vi "RMX410x Configuration.vi"() -> ()   [LabVIEW 2019]
uses:
  <vilib>/addons/VeriStand Custom Device Scripting APIs/Instrument Addon/Libraries Directory/Protocols.lvlibp/RS-xxx/RS-xxx Settings.ctl
  <vilib>/addons/VeriStand Custom Device Scripting APIs/Instrument Addon/API/TypeDefs/Message Settings.ctl
  <vilib>/addons/VeriStand Custom Device Scripting APIs/Instrument Addon/API/TypeDefs/Protection Types.ctl
  <vilib>/NI VeriStand/Custom Device API/Custom Device Item Ref.ctl
  <vilib>/addons/VeriStand Custom Device Scripting APIs/Instrument Addon/API/TypeDefs/Single Channel Enumerated List Settings.ctl
  <vilib>/addons/VeriStand Custom Device Scripting APIs/Instrument Addon/API/TypeDefs/Single Channel Format Settings.ctl
  <vilib>/addons/VeriStand Custom Device Scripting APIs/Instrument Addon/API/TypeDefs/Command Settings.ctl
  <vilib>/addons/VeriStand Custom Device Scripting APIs/Instrument Addon/API/TypeDefs/Padding.ctl
  <vilib>/addons/VeriStand Custom Device Scripting APIs/Instrument Addon/API/TypeDefs/ByteCount Response Settings.ctl
  <vilib>/addons/VeriStand Custom Device Scripting APIs/Instrument Addon/API/TypeDefs/Linked Channel.ctl
  <vilib>/addons/VeriStand Custom Device Scripting APIs/Instrument Addon/API/Messages/Create Message - Periodic & Trigger.vi
  <vilib>/addons/VeriStand Custom Device Scripting APIs/Instrument Addon/API/Messages/Configure Response - Byte Count.vi
  <vilib>/addons/VeriStand Custom Device Scripting APIs/Instrument Addon/API/Messages/Create Message - Value Change & Trigger.vi
  <vilib>/addons/VeriStand Custom Device Scripting APIs/Instrument Addon/API/Channels/Create MetaData Channel - Single Channel - Format.vi
  <vilib>/addons/VeriStand Custom Device Scripting APIs/Instrument Addon/API/Channels/Create MetaData Channel - Single Channel - Enumerated List.vi
  <vilib>/addons/VeriStand Custom Device Scripting APIs/Instrument Addon/API/Channels/Create Data Channel - Single Channel - Enumerated List.vi
  <vilib>/addons/VeriStand Custom Device Scripting APIs/Instrument Addon/API/Custom Device/RS-xxx Factory.vi
  <vilib>/addons/VeriStand Custom Device Scripting APIs/Instrument Addon/API/Channels/Create Data Channel - Single Channel - Format.vi
  <vilib>/addons/VeriStand Custom Device Scripting APIs/Instrument Addon/API/Instrument Addon Scripting API.lvlib
  <vilib>/addons/VeriStand Custom Device Scripting APIs/Instrument Addon/Libraries Directory/Protocols.lvlibp/RS-xxx/RS-xxx.lvclass
  <vilib>/NI VeriStand/Custom Device API/Custom Device API.lvlib
panel:
  in  "Output System Definition File":path=path "System Definition Files/RMX410x Scripted.nivssdf"
  in  "Input System Definition File":path=path "System Definition Files/Base.nivssdf"
  # "Overview: Creates an Instrument Addon Custom Device and adds the messages and channels used to operate the NI RMX410x Rackmount Programmable DC Power Supply.\n\nThe VI executes the following steps:\n1. Creates a new Instrument Addon in the target system definition file with an RS-xxx protocol type.\n2. Creates Configuration, Control, and Feedback groups.\n3. Configures messages with created MetaData and Data Channels.\n4. Configures the messages for controlling and getting feedback from the RMX410x device.\n5. Configures the channels that control the output state and voltage levels.\n\nInstructions:\n1. Browse to the system definition file to be used as input.\n2. Browse to a path to save the system definition file as output. This may be the same as the input file.\n3. Run the VI and verify its results. \n\nFor more information on the RMX410x, refer to the RMX410x User manual:\nhttps://www.ni.com/pdf/manuals/377396c.pdf)"
  # "System Definition Files"
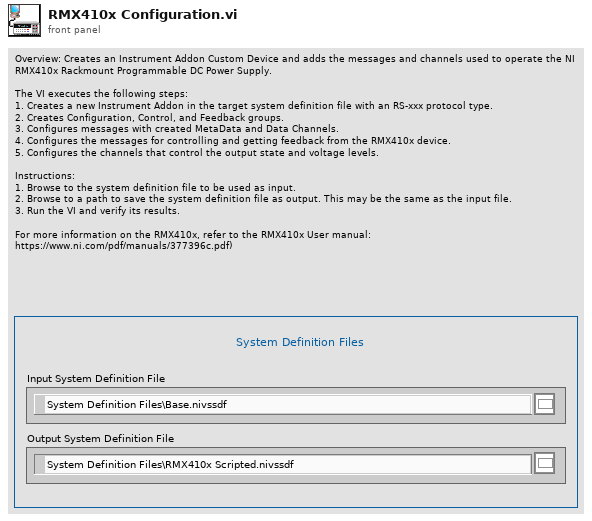
[diagram p1: front panel]
types:
  T1 = typedef "Instrument Addon Scripting API.lvlib/Linked Channel.ctl" = cluster{"Variable Name":string, "Channel Refnum":T2}
  T2 = typedef "Custom Device API.lvlib/Custom Device Item Ref.ctl" = u64
  T3 = typedef "Instrument Addon Scripting API.lvlib/ByteCount Response Settings.ctl" = cluster{"Response Format":string, "Linked Channels":T1[], "Byte Count":i32, "Use Byte Count channel":bool, "Channel Refnum":T2}
  T4 = typedef "Instrument Addon Scripting API.lvlib/Single Channel Format Settings.ctl" = cluster{"Format String":string, "Default Value":dbl, "Units":string}
  T5 = typedef "Instrument Addon Scripting API.lvlib/Single Channel Enumerated List Settings.ctl" = cluster{"Enumerated List":string[], "Default Value":dbl, "Units":string}
  T6 = cluster{"Variable Name":string, "Channel Ref in":T2}
  T7 = typedef "Instrument Addon Scripting API.lvlib/Command Settings.ctl" = cluster{"Command Format":string, "Linked Channels":cluster{"Variable Name":string, "Channel Ref in":T2}[], "Use Padding?":bool, "Padding":T8}
  T8 = typedef "Instrument Addon Scripting API.lvlib/Padding.ctl" = cluster{"Pad Value":u8, "Length":u32}
  T9 = typedef "Instrument Addon Scripting API.lvlib/Protection Types.ctl" = enum16{"None", "CRC-32", "Checksum U16", "Checksum U32", "Checksum U8"}
  T10 = typedef "Instrument Addon Scripting API.lvlib/Message Settings.ctl" = cluster{"Protection":T9, "Enable Periodic Default":bool, "Trigger Channel refnum":u64}
  T11 = enum16{"NUL", "SOH", "STX", "ETX", "EOT", "ENQ", "ACK", "BEL", "BS", "HT", "LF", "VT", "FF", "CR", "SO", "SI", "DLE", "DC1", "DC2", "DC3", "DC4", "NAK", "SYN", "ETB", "CAN", "EM", "SUB", "ESC", "FS", "GS", "RS", "US", "SP", "!", "\"", "#", "$", "%", "&", "'", "(", ")", "*", "+", ",", "- (-)", ".", "/", "0", "1", "2", "3", "4", "5", "6", "7", "8", "9", ":", ";", "<", "=", ">", "?", "@", "A", "B", "C", "D", "E", "F", "G", "H", "I", "J", "K", "L", "M", "N", "O", "P", "Q", "R", "S", "T", "U", "V", "W", "X", "Y", "Z", "[", "\\", "]", "^", "_", "`", "a", "b", "c", "d", "e", "f", "g", "h", "i", "j", "k", "l", "m", "n", "o", "p", "q", "r", "s", "t", "u", "v", "w", "x", "y", "z", "{", "|", "}", "~"}
  T12 = typedef "Protocols.lvlibp/RS-xxx.lvclass/RS-xxx Settings.ctl" = cluster{"Port":string, "Baud Rate":u32, "Data Bits":u16, "Parity":enum16{"None", "Odd", "Even", "Mark", "Space"}, "Stop Bits":u16, "Flow Control":u16, "XON":enum16{"NUL", "SOH", "STX", "ETX", "EOT", "ENQ", "ACK", "BEL", "BS", "HT", "LF", "VT", "FF", "CR", "SO", "SI", "DLE", "DC1", "DC2", "DC3", "DC4", "NAK", "SYN", "ETB", "CAN", "EM", "SUB", "ESC", "FS", "GS", "RS", "US", "SP", "!", "\"", "#", "$", "%", "&", "'", "(", ")", "*", "+", ",", "- (-)", ".", "/", "0", "1", "2", "3", "4", "5", "6", "7", "8", "9", ":", ";", "<", "=", ">", "?", "@", "A", "B", "C", "D", "E", "F", "G", "H", "I", "J", "K", "L", "M", "N", "O", "P", "Q", "R", "S", "T", "U", "V", "W", "X", "Y", "Z", "[", "\\", "]", "^", "_", "`", "a", "b", "c", "d", "e", "f", "g", "h", "i", "j", "k", "l", "m", "n", "o", "p", "q", "r", "s", "t", "u", "v", "w", "x", "y", "z", "{", "|", "}", "~"}, "XOFF":enum16{"NUL", "SOH", "STX", "ETX", "EOT", "ENQ", "ACK", "BEL", "BS", "HT", "LF", "VT", "FF", "CR", "SO", "SI", "DLE", "DC1", "DC2", "DC3", "DC4", "NAK", "SYN", "ETB", "CAN", "EM", "SUB", "ESC", "FS", "GS", "RS", "US", "SP", "!", "\"", "#", "$", "%", "&", "'", "(", ")", "*", "+", ",", "- (-)", ".", "/", "0", "1", "2", "3", "4", "5", "6", "7", "8", "9", ":", ";", "<", "=", ">", "?", "@", "A", "B", "C", "D", "E", "F", "G", "H", "I", "J", "K", "L", "M", "N", "O", "P", "Q", "R", "S", "T", "U", "V", "W", "X", "Y", "Z", "[", "\\", "]", "^", "_", "`", "a", "b", "c", "d", "e", "f", "g", "h", "i", "j", "k", "l", "m", "n", "o", "p", "q", "r", "s", "t", "u", "v", "w", "x", "y", "z", "{", "|", "}", "~"}, "End Read on Termination Character":bool, "End Write on Termination Character":bool, "Termination Character":u8}
  T13 = cluster{"Variable Name":string, "Channel Ref in":T2}[]
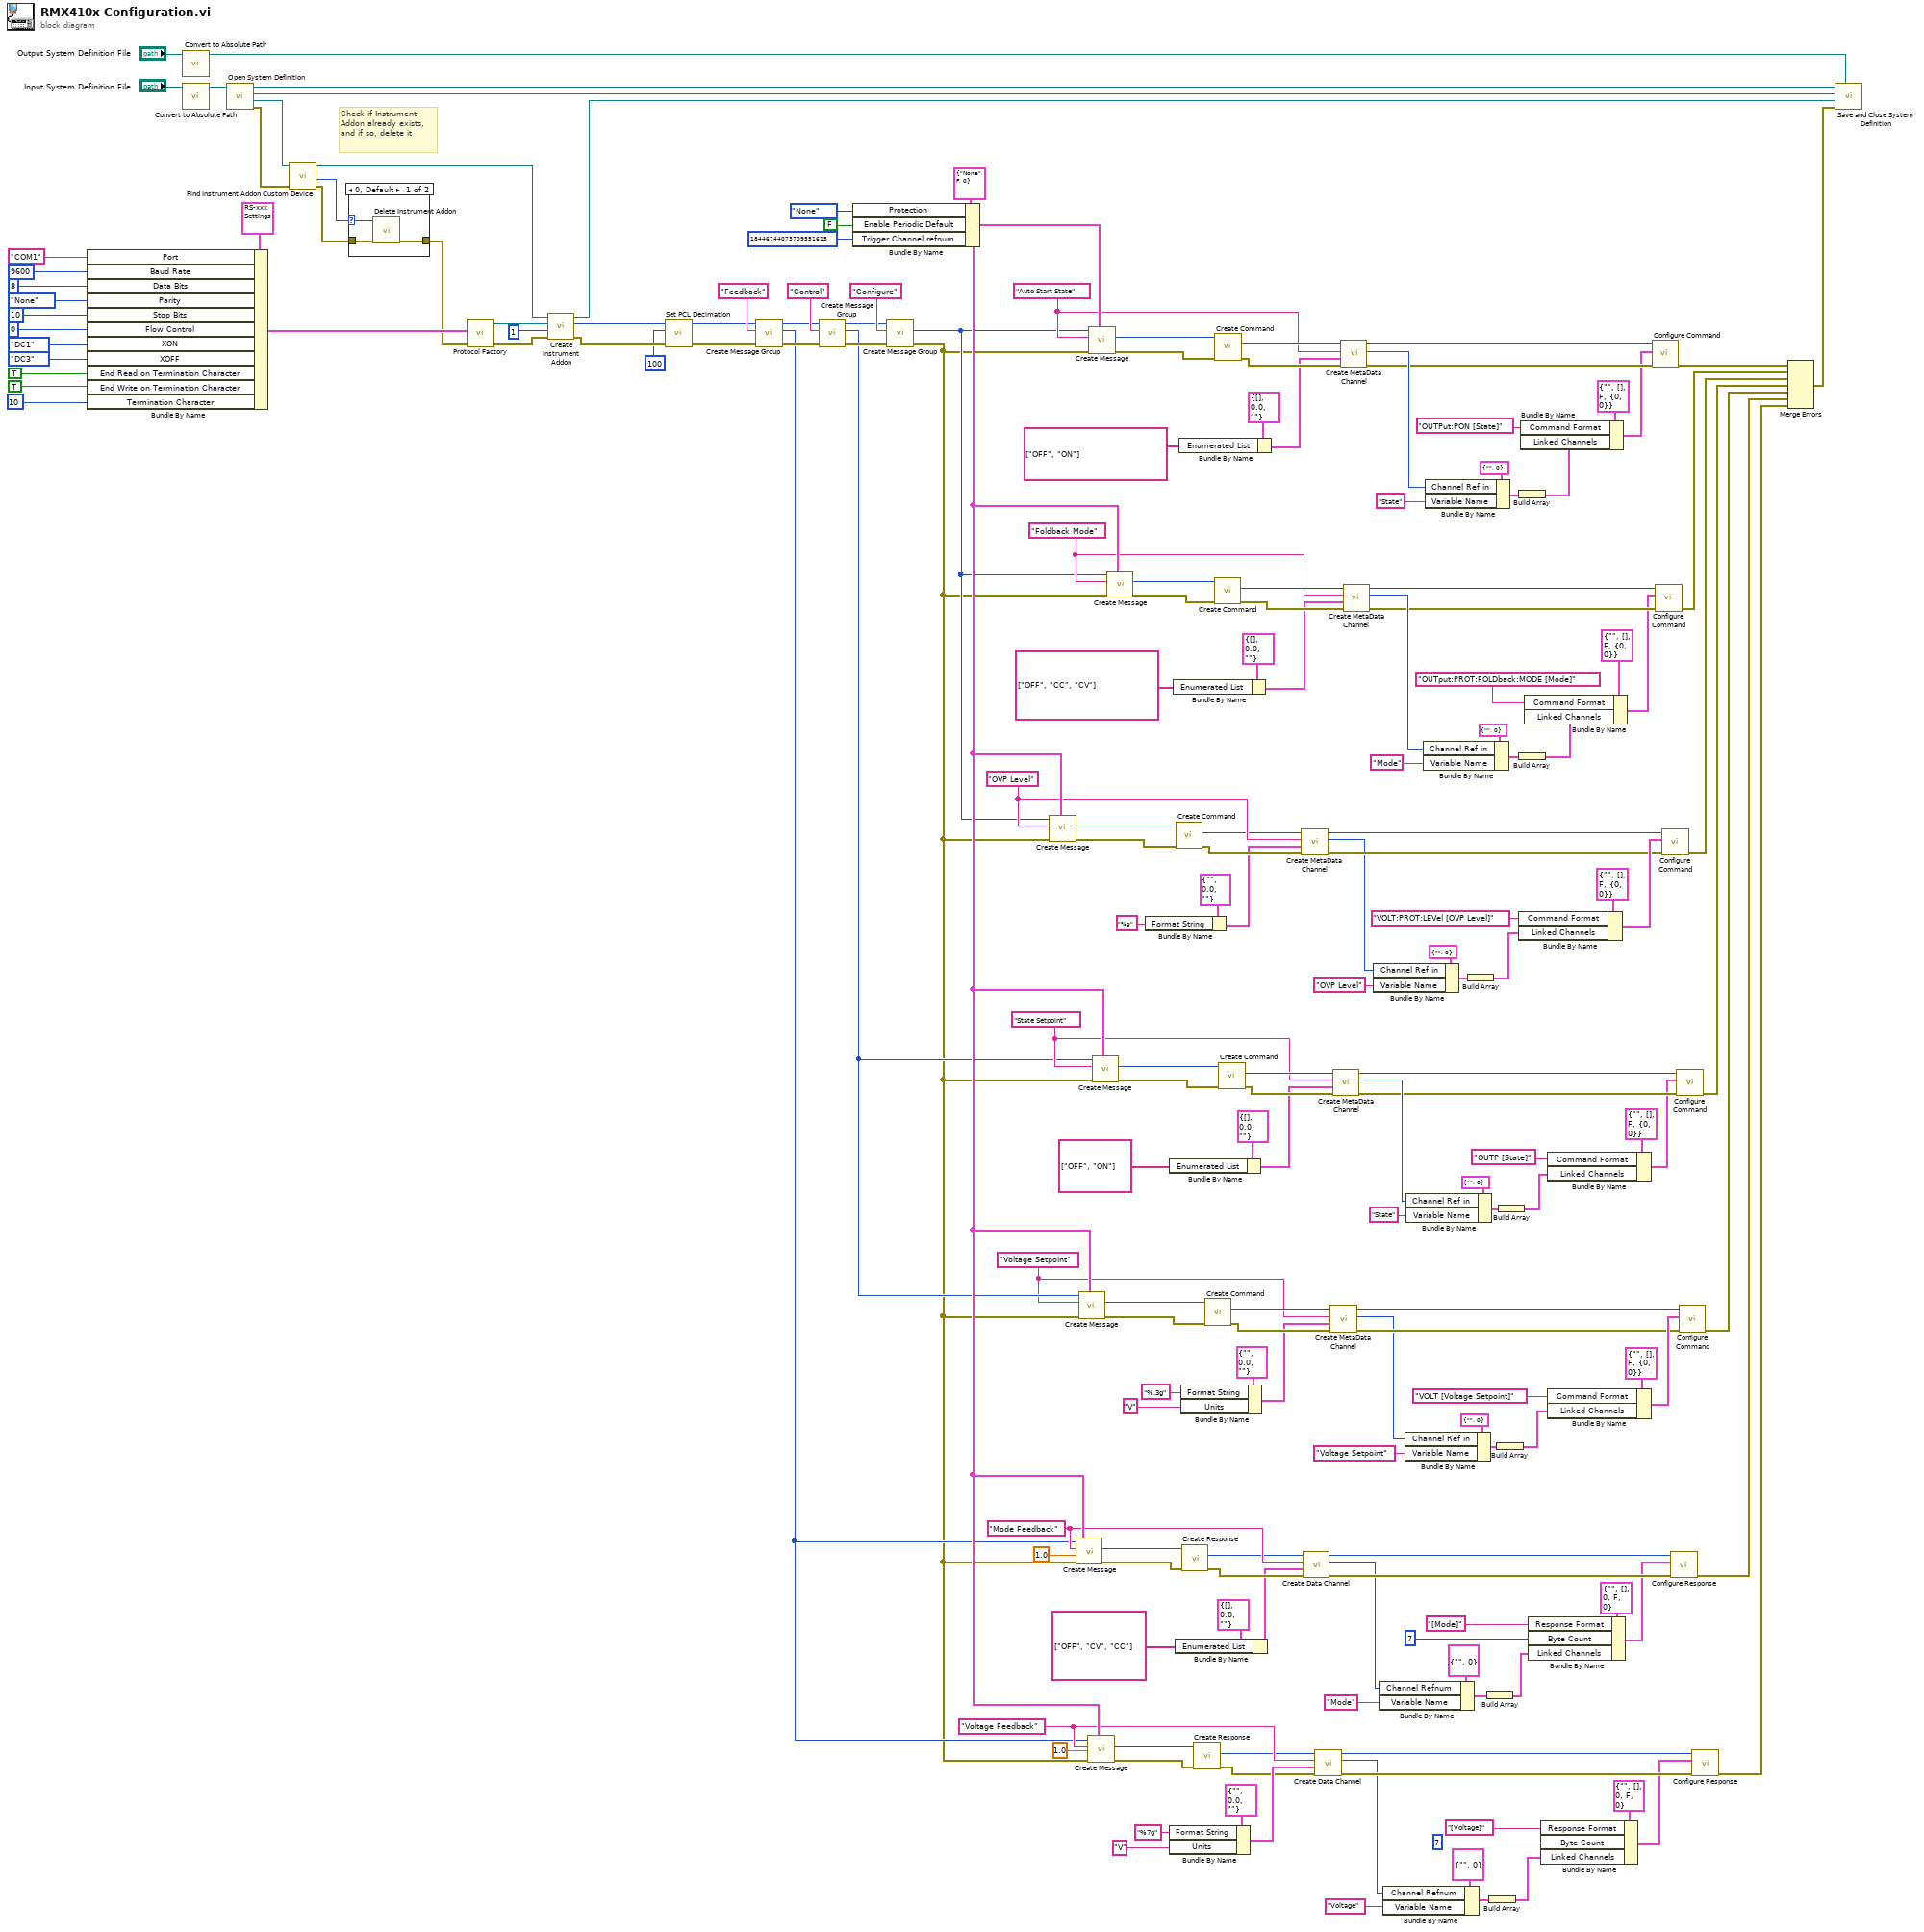
[diagram p0: block diagram]
diagram:
  w24 = "Voltage Feedback" ("message name")
  w47 = "Mode Feedback" ("message name")
  w65 = "Voltage Setpoint" ("message name")
  w85 = "State Setpoint" ("message name")
  w124 = "OVP Level" ("message name")
  w127 = "Foldback Mode" ("message name")
  w126 = "Auto Start State" ("message name")
  # "Check if Instrument Addon already exists, and if so, delete it"
  n1 = Bundle By Name(cluster=T12 {"Port"="", "Baud Rate"=0, "Data Bits"=0, "Parity"=enum."None", "Stop Bits"=0, "Flow Control"=0, "XON"=enum."NUL", "XOFF"=enum."NUL", "End Read on Termination Character"=FALSE, "End Write on Termination Character"=FALSE, "Termination Character"=0} ("RS-xxx settings"), "Port"="COM1", "Baud Rate"=u32 9600, "Data Bits"=u16 8, "Parity"=enum16{"None", "Odd", "Even", "Mark", "Space"}."None", "Stop Bits"=u16 10, "Flow Control"=u16 0, "XON"=T11."DC1", "XOFF"=T11."DC3", "End Read on Termination Character"=TRUE, "End Write on Termination Character"=TRUE ("End Read on Termination Character"), "Termination Character"=u8 10) -> (w187:T12)
  n2 = call "Convert to Absolute Path.vi"("System Definition File"="Output System Definition File") -> ("Absolute Path"=w1:path)  [unwired: 10 in]
  n3 = call "Convert to Absolute Path.vi"("System Definition File"="Input System Definition File") -> ("Absolute Path"=w8:path)  [unwired: 10 in]
  n4 = call "Open System Definition.vi"("System Definition File"=w8) -> ("error out"=w172:errorcluster, "Target Refnum"=w173:refnum<k24>, "Root Refnum"=w4:refnum<k24>, "System Definition Refnum"=w5:refnum<k24>)  [unwired: 7 in]
  n5 = call "Find Instrument Addon Custom Device.vi"("error in"=w172, "target in"=w173) -> ("error out"=w171:errorcluster, "NodeID"=w153:u64, "target out"=w169:refnum<k24>)  [unwired: 7 in]
  n6 = case shown="0, Default" w153 {
    selector: w153 -> [w191 _]
    tunnel: w171 -> [w193 w194]
    tunnel: [w192 w194] -> w170
    frame 0, Default {
      n7 = call <vilib>:"Delete Instrument Addon.vi"("error in (no error)"=w193, "instrument addon refnum"=w191) -> ("error out"=w192:errorcluster)  [unwired: 9 in]
    }
    frame -1 {
    }
  }
  n8 = call-poly <vilib>:"Protocol Factory.vi"("error in (no error)"=w170, "settings"=w187) -> ("error out"=w174:errorcluster, "protocol out"=w189:refnum<class "Protocol Parent.lvclass">)  [unwired: 8 in]
  n9 = call <vilib>:"Create Instrument Addon.vi"("error in (no error)"=w174, "PCL decimation"=u16 1, "protocol in"=w189, "target in"=w169) -> ("error out"=w15:errorcluster, "instrument addon refnum"=w16:T2, "target out"=w3:refnum<k24>)  [unwired: 5 in]
  n10 = call <vilib>:"Set PCL Decimation.vi"("error in (no error)"=w15, "PCL decimation"=u32 100, "instrument addon refnum in"=w16) -> ("error out"=w13:errorcluster, "instrument addon refnum"=w14:T2)  [unwired: 7 in]
  n11 = call <vilib>:"Create Message Group.vi"("error in (no error)"=w13, "message group name"="Feedback", "instrument addon refnum in"=w14) -> ("error out"=w102:errorcluster, "message group refnum out"=w19:T2, "instrument addon refnum out"=w103:T2)  [unwired: 6 in]
  n12 = call <vilib>:"Create Message Group.vi"("error in (no error)"=w102, "message group name"="Control", "instrument addon refnum in"=w103) -> ("error out"=w100:errorcluster, "message group refnum out"=w66:T2, "instrument addon refnum out"=w101:T2)  [unwired: 6 in]
  n13 = Bundle By Name(cluster=T10 {"Protection"=enum."None", "Enable Periodic Default"=FALSE, "Trigger Channel refnum"=0} ("optional settings"), "Protection"=Protection_Types."None", "Enable Periodic Default"=FALSE, "Trigger Channel refnum"=T2 18446744073709551615 ("command refnum")) -> (w190:T10)
  n14 = call <vilib>:"Create Message Group.vi"("error in (no error)"=w100, "message group name"="Configure", "instrument addon refnum in"=w101) -> ("error out"=w11:errorcluster, "message group refnum out"=w81:T2)  [unwired: 6 in, 1 out]
  n15 = call-poly <vilib>:"Create Message.vi"("optional settings"=w190, "error in (no error)"=w11, "message name"=w124, "message group refnum in"=w81) -> ("error out"=w111:errorcluster, "message refnum out"=w110:T2)  [unwired: 5 in, 1 out]
  n16 = call-poly <vilib>:"Create Message.vi"("optional settings"=w190, "error in (no error)"=w11, "period (s)"=1.0, "message name"=w47, "message group refnum in"=w19) -> ("error out"=w44:errorcluster, "message refnum out"=w43:T2)  [unwired: 4 in, 1 out]
  n17 = call-poly <vilib>:"Create Message.vi"("optional settings"=w190, "error in (no error)"=w11, "message name"=w65, "message group refnum in"=w66) -> ("error out"=w68:errorcluster, "message refnum out"=w67:T2)  [unwired: 5 in, 1 out]
  n18 = call-poly <vilib>:"Create Message.vi"("optional settings"=w190, "error in (no error)"=w11, "period (s)"=1.0, "message name"=w24, "message group refnum in"=w19) -> ("error out"=w21:errorcluster, "message refnum out"=w20:T2)  [unwired: 4 in, 1 out]
  n19 = call-poly <vilib>:"Create Message.vi"("optional settings"=w190, "error in (no error)"=w11, "message name"=w126, "message group refnum in"=w81) -> ("error out"=w166:errorcluster, "message refnum out"=w167:T2)  [unwired: 5 in, 1 out]
  n20 = call-poly <vilib>:"Create Message.vi"("optional settings"=w190, "error in (no error)"=w11, "message name"=w85, "message group refnum in"=w66) -> ("error out"=w98:errorcluster, "message refnum out"=w99:T2)  [unwired: 5 in, 1 out]
  n21 = call-poly <vilib>:"Create Message.vi"("optional settings"=w190, "error in (no error)"=w11, "message name"=w127, "message group refnum in"=w81) -> ("error out"=w143:errorcluster, "message refnum out"=w144:T2)  [unwired: 5 in, 1 out]
  n22 = Bundle By Name(cluster=T4 {"Format String"="", "Default Value"=0.0, "Units"=""} ("settings"), "Format String"="%g") -> (w108:T4)
  n23 = Bundle By Name(cluster=T5 {"Enumerated List"=[], "Default Value"=0.0, "Units"=""} ("settings"), "Enumerated List"=string[] ["OFF", "ON"]) -> (w83:T5)
  n24 = Bundle By Name(cluster=T4 {"Format String"="", "Default Value"=0.0, "Units"=""} ("settings"), "Format String"="%7g", "Units"="V") -> (w26:T4)
  n25 = Bundle By Name(cluster=T5 {"Enumerated List"=[], "Default Value"=0.0, "Units"=""} ("settings"), "Enumerated List"=string[] ["OFF", "CC", "CV"]) -> (w138:T5)
  n26 = Bundle By Name(cluster=T5 {"Enumerated List"=[], "Default Value"=0.0, "Units"=""} ("settings"), "Enumerated List"=string[] ["OFF", "CV", "CC"]) -> (w41:T5)
  n27 = call <vilib>:"Create Command.vi"("error in"=w111, "message refnum In"=w110) -> ("error out"=w113:errorcluster, "command refnum"=w112:T2)  [unwired: 7 in, 1 out]
  n28 = Bundle By Name(cluster=T5 {"Enumerated List"=[], "Default Value"=0.0, "Units"=""} ("settings"), "Enumerated List"=string[] ["OFF", "ON"]) -> (w161:T5)
  n29 = Bundle By Name(cluster=T4 {"Format String"="", "Default Value"=0.0, "Units"=""} ("settings"), "Format String"="%.3g", "Units"="V") -> (w63:T4)
  n30 = call <vilib>:"Create Response.vi"("error in (no error)"=w44, "message refnum in"=w43) -> ("error out"=w46:errorcluster, "response refnum"=w45:T2)  [unwired: 7 in, 1 out]
  n31 = call <vilib>:"Create Response.vi"("error in (no error)"=w21, "message refnum in"=w20) -> ("error out"=w23:errorcluster, "response refnum"=w22:T2)  [unwired: 7 in, 1 out]
  n32 = call <vilib>:"Create Command.vi"("error in"=w68, "message refnum In"=w67) -> ("error out"=w70:errorcluster, "command refnum"=w69:T2)  [unwired: 7 in, 1 out]
  n33 = call <vilib>:"Create Command.vi"("error in"=w143, "message refnum In"=w144) -> ("error out"=w141:errorcluster, "command refnum"=w142:T2)  [unwired: 7 in, 1 out]
  n34 = call <vilib>:"Create Command.vi"("error in"=w166, "message refnum In"=w167) -> ("error out"=w164:errorcluster, "command refnum"=w165:T2)  [unwired: 7 in, 1 out]
  n35 = call <vilib>:"Create Command.vi"("error in"=w98, "message refnum In"=w99) -> ("error out"=w96:errorcluster, "command refnum"=w97:T2)  [unwired: 7 in, 1 out]
  n36 = call-poly <vilib>:"Create MetaData Channel.vi"("error in (no error)"=w113, "settings"=w108, "channel name"=w124, "command refnum in"=w112) -> ("error out"=w116:errorcluster, "channel refnum"=w115:T2, "command refnum out"=w114:T2)  [unwired: 5 in]
  n37 = call-poly <vilib>:"Create Data Channel.vi"("error in (no error)"=w46, "settings"=w41, "channel name"=w47, "response refnum in"=w45) -> ("error out"=w58:errorcluster, "channel refnum"=w53:T2, "response refnum out"=w48:T2)  [unwired: 5 in]
  n38 = call-poly <vilib>:"Create Data Channel.vi"("error in (no error)"=w23, "settings"=w26, "channel name"=w24, "response refnum in"=w22) -> ("error out"=w39:errorcluster, "channel refnum"=w34:T2, "response refnum out"=w29:T2)  [unwired: 5 in]
  n39 = call-poly <vilib>:"Create MetaData Channel.vi"("error in (no error)"=w70, "settings"=w63, "channel name"=w65, "command refnum in"=w69) -> ("error out"=w73:errorcluster, "channel refnum"=w72:T2, "command refnum out"=w71:T2)  [unwired: 5 in]
  n40 = call-poly <vilib>:"Create MetaData Channel.vi"("error in (no error)"=w96, "settings"=w83, "channel name"=w85, "command refnum in"=w97) -> ("error out"=w93:errorcluster, "channel refnum"=w94:T2, "command refnum out"=w95:T2)  [unwired: 5 in]
  n41 = call-poly <vilib>:"Create MetaData Channel.vi"("error in (no error)"=w164, "settings"=w161, "channel name"=w126, "command refnum in"=w165) -> ("error out"=w158:errorcluster, "channel refnum"=w159:T2, "command refnum out"=w160:T2)  [unwired: 5 in]
  n42 = call-poly <vilib>:"Create MetaData Channel.vi"("error in (no error)"=w141, "settings"=w138, "channel name"=w127, "command refnum in"=w142) -> ("error out"=w135:errorcluster, "channel refnum"=w136:T2, "command refnum out"=w137:T2)  [unwired: 5 in]
  n43 = Bundle By Name(cluster=T6 {"Variable Name"="", "Channel Ref in"=0} ("Linked Channel"), "Channel Ref in"=w115, "Variable Name"="OVP Level") -> (w121:T6)
  n44 = Bundle By Name(cluster=T1 {"Variable Name"="", "Channel Refnum"=0} ("Linked Channel"), "Channel Refnum"=w53, "Variable Name"="Mode") -> (w55:T1)
  n45 = Bundle By Name(cluster=T1 {"Variable Name"="", "Channel Refnum"=0} ("Linked Channel"), "Channel Refnum"=w34, "Variable Name"="Voltage") -> (w36:T1)
  n46 = Bundle By Name(cluster=T6 {"Variable Name"="", "Channel Ref in"=0} ("Linked Channel"), "Channel Ref in"=w72, "Variable Name"="Voltage Setpoint") -> (w78:T6)
  n47 = Bundle By Name(cluster=T6 {"Variable Name"="", "Channel Ref in"=0} ("Linked Channel"), "Channel Ref in"=w94, "Variable Name"="State") -> (w88:T6)
  n48 = Bundle By Name(cluster=T6 {"Variable Name"="", "Channel Ref in"=0} ("Linked Channel"), "Channel Ref in"=w136, "Variable Name"="Mode") -> (w130:T6)
  n49 = Bundle By Name(cluster=T6 {"Variable Name"="", "Channel Ref in"=0} ("Linked Channel"), "Channel Ref in"=w159, "Variable Name"="State") -> (w148:T6)
  n50 = Build Array(w121) -> (w122:T13)
  n51 = Build Array(w55) -> (w56:T1[])
  n52 = Build Array(w36) -> (w37:T1[])
  n53 = Build Array(w78) -> (w79:T13)
  n54 = Build Array(w88) -> (w87:T13)
  n55 = Build Array(w148) -> (w147:T13)
  n56 = Build Array(w130) -> (w129:T13)
  n57 = Bundle By Name(cluster=T7 {"Command Format"="", "Linked Channels"=[], "Use Padding?"=FALSE, "Padding"={"Pad Value"=0, "Length"=0}} ("settings"), "Command Format"="VOLT:PROT:LEVel [OVP Level]", "Linked Channels"=w122) -> (w123:T7)
  n58 = Bundle By Name(cluster=T7 {"Command Format"="", "Linked Channels"=[], "Use Padding?"=FALSE, "Padding"={"Pad Value"=0, "Length"=0}} ("settings"), "Command Format"="OUTPut:PON [State]", "Linked Channels"=w147) -> (w146:T7)
  n59 = Bundle By Name(cluster=T7 {"Command Format"="", "Linked Channels"=[], "Use Padding?"=FALSE, "Padding"={"Pad Value"=0, "Length"=0}} ("settings"), "Command Format"="OUTput:PROT:FOLDback:MODE [Mode]", "Linked Channels"=w129) -> (w128:T7)
  n60 = Bundle By Name(cluster=T3 {"Response Format"="", "Linked Channels"=[], "Byte Count"=0, "Use Byte Count channel"=FALSE, "Channel Refnum"=0} ("settings"), "Response Format"="[Mode]", "Byte Count"=7, "Linked Channels"=w56) -> (w51:T3)
  n61 = Bundle By Name(cluster=T3 {"Response Format"="", "Linked Channels"=[], "Byte Count"=0, "Use Byte Count channel"=FALSE, "Channel Refnum"=0} ("settings"), "Response Format"="[Voltage]", "Byte Count"=7, "Linked Channels"=w37) -> (w32:T3)
  n62 = Bundle By Name(cluster=T7 {"Command Format"="", "Linked Channels"=[], "Use Padding?"=FALSE, "Padding"={"Pad Value"=0, "Length"=0}} ("settings"), "Command Format"="OUTP [State]", "Linked Channels"=w87) -> (w86:T7)
  n63 = Bundle By Name(cluster=T7 {"Command Format"="", "Linked Channels"=[], "Use Padding?"=FALSE, "Padding"={"Pad Value"=0, "Length"=0}} ("settings"), "Command Format"="VOLT [Voltage Setpoint]", "Linked Channels"=w79) -> (w80:T7)
  n64 = call <vilib>:"Configure Command.vi"("error in (no error)"=w158, "settings"=w146, "command refnum in"=w160) -> ("error out"=w145:errorcluster)  [unwired: 7 in, 1 out]
  n65 = call <vilib>:"Configure Command.vi"("error in (no error)"=w135, "settings"=w128, "command refnum in"=w137) -> ("error out"=w125:errorcluster)  [unwired: 7 in, 1 out]
  n66 = call <vilib>:"Configure Command.vi"("error in (no error)"=w116, "settings"=w123, "command refnum in"=w114) -> ("error out"=w106:errorcluster)  [unwired: 7 in, 1 out]
  n67 = call-poly <vilib>:"Configure Response.vi"("error in (no error)"=w58, "settings"=w51, "response refnum in"=w48) -> ("error out"=w17:errorcluster)  [unwired: 7 in, 1 out]
  n68 = call <vilib>:"Configure Command.vi"("error in (no error)"=w93, "settings"=w86, "command refnum in"=w95) -> ("error out"=w61:errorcluster)  [unwired: 7 in, 1 out]
  n69 = call <vilib>:"Configure Command.vi"("error in (no error)"=w73, "settings"=w80, "command refnum in"=w71) -> ("error out"=w59:errorcluster)  [unwired: 7 in, 1 out]
  n70 = call-poly <vilib>:"Configure Response.vi"("error in (no error)"=w39, "settings"=w32, "response refnum in"=w29) -> ("error out"=w18:errorcluster)  [unwired: 7 in, 1 out]
  n71 = Merge Errors(w145, w125, w106, w61, w59, w17, w18) -> (w2:errorcluster)
  n72 = call "Save and Close System Definition.vi"("System Definition Path"=w1, "error in (no error)"=w2, "Target Refnum"=w3, "Root Refnum"=w4, "System Definition Refnum"=w5) -> ()  [unwired: 6 in, 1 out]
